vi "Command Type.vi"(11 "Error Command Config in":refnum<class "Error Command Config.lvclass">) -> (2 "Command Type":T1)   [LabVIEW 2020, in "VolatusSeqConfig.lvlib" / "Error Command Config.lvclass"]
uses:
  Error Command Config.lvclass
  Error Command Config.lvclass/Error Command Config.ctl
  Command Type.ctl
  VolatusSeqConfig.lvlib
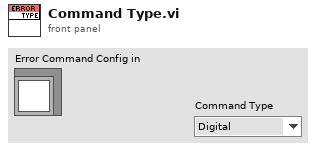
[diagram p1: front panel]
types:
  T1 = typedef "VolatusSeqConfig.lvlib/Command Type.ctl" = enum16{"Digital", "Numeric", "Transition", "Stop", "StartLog", "StopLog", "Start", "Event", "Error", "HTTP"}
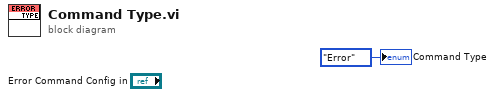
[diagram p0: block diagram]
diagram:
  "Command Type" <- Command_Type."Error" ("Command Type")
